vi "class_data.vi"() -> ()   [LabVIEW 2010, in "Image.lvclass"]
uses:
  Image.lvclass
panel:
  out "temp file folder":path
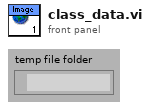
[diagram p1: front panel]
diagram:
